vi "Calculate Power, PP, F@PP, V@PP.vi"(10 "Velocity Array":dbl[](array[numeric]), 11 "Force Array":dbl[](array[numeric])) -> (1 "Force at PP":dbl, 2 "Peak Power":dbl, 3 "Power Array":dbl[](array[numeric]), 4 "Velocity at PP":dbl)   [LabVIEW 2016]
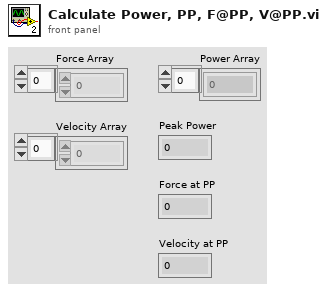
[diagram p1: front panel]
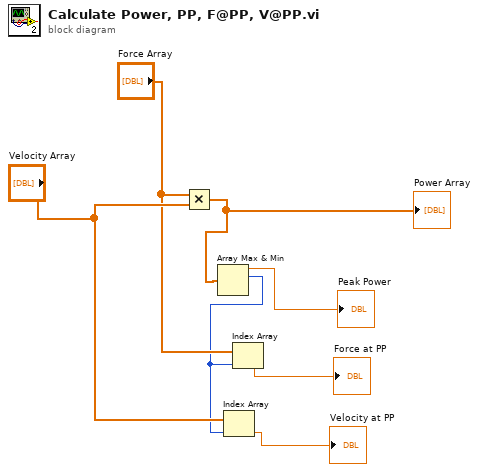
[diagram p0: block diagram]
diagram:
  n1 = Multiply(x="Force Array", y="Velocity Array") -> (x*y=w1:dbl[])
  "Power Array" <- w1
  n2 = Array Max & Min(array=w1) -> (max value=→"Peak Power":dbl, max index (indices)=w4:i32)  [unwired: 2 out]
  n3 = Index Array "Index Array"(array="Velocity Array", index=w4) -> (element=→"Velocity at PP":dbl)
  n4 = Index Array "Index Array"(array="Force Array", index=w4) -> (element=→"Force at PP":dbl)
